vi "Toggle.vi"() -> ()   [LabVIEW 2019]
panel:
  out "Toggled Output":bool
  in  "Input":bool=TRUE
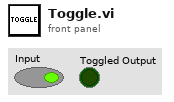
[diagram p1: front panel]
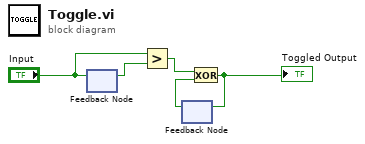
[diagram p0: block diagram]
diagram:
  n1 = feedback #1() -> (w3:bool)  [unwired: 1 in]
  n2 = feedback-in #1("Input") -> ()
  n3 = Greater?(x="Input", y=w3) -> (0:w5:bool)
  n4 = feedback #2() -> (w4:bool)  [unwired: 1 in]
  n5 = Exclusive Or(1:w4, 2:w5) -> (0:w2:bool)
  "Toggled Output" <- w2
  n6 = feedback-in #2(w2) -> ()
